vi "LoadUserInterface.vi"(8 "error in (no error)":errorcluster, 10 "Actor In":refnum<class "Actor.lvclass">, 11 "QuickNote in":refnum<class "QuickNote.lvclass">) -> (0 "error out":errorcluster, 3 "QuickNote out":refnum<class "QuickNote.lvclass">)   [LabVIEW 2020, in "QuickNote.lvlib" / "QuickNote.lvclass"]
uses:
  QuickNote.lvclass
  <vilib>/ActorFramework/Actor/Actor.lvclass
  QuickNoteUI/QuickNoteUI.lvclass
  C:/Program Files/National Instruments/LabVIEW 2020/vi.lib/ActorFramework/Actor/Actor.lvclass
  DataProcessor/DataProcessor/DataProcessor.lvclass
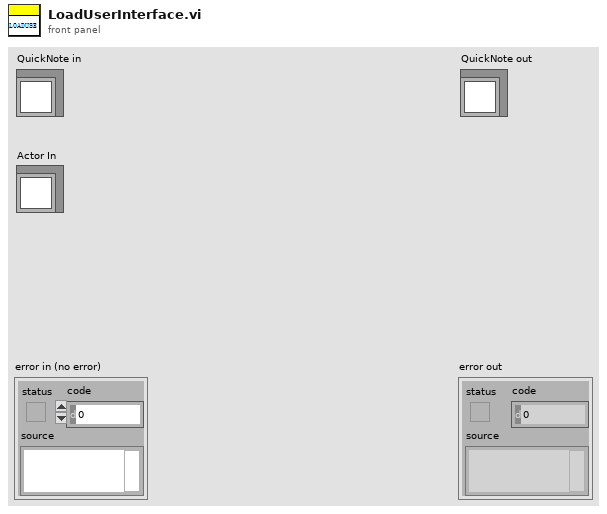
[diagram p1: front panel]
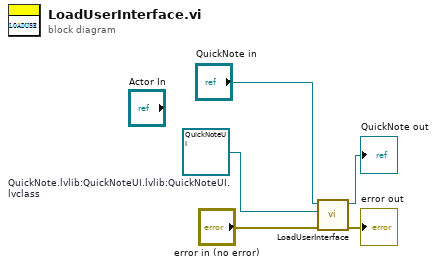
[diagram p0: block diagram]
diagram:
  w1 = refnum<class "QuickNoteUI.lvclass"> refnum  # QuickNote.lvlib:QuickNoteUI.lvlib:QuickNoteUI.lvclass
  n1 = call-parent "LoadUserInterface.vi"("error in (no error)"="error in (no error)", "Actor In"=w1, "DataProcessor in"="QuickNote in") -> ("error out"=→"error out":errorcluster, "DataProcessor out"=→"QuickNote out":refnum<class "QuickNote.lvclass">)  [unwired: 7 in]
